vi "故障告警分析.vi"(8 "告警代码":u16, 9 "故障代码":u16, 10 "运行步序":u16, 11 "参数":string) -> (2 "报警内容":T1, 3 "简易报警状态":cluster{"故障状态":string, "报警状态":string})   [LabVIEW 2016, in "斯坦道氨氮.lvlib"]
panel:
  # "1、注射泵水样阀口堵塞；\n2、注射泵阀过载或丝杆无动作。"
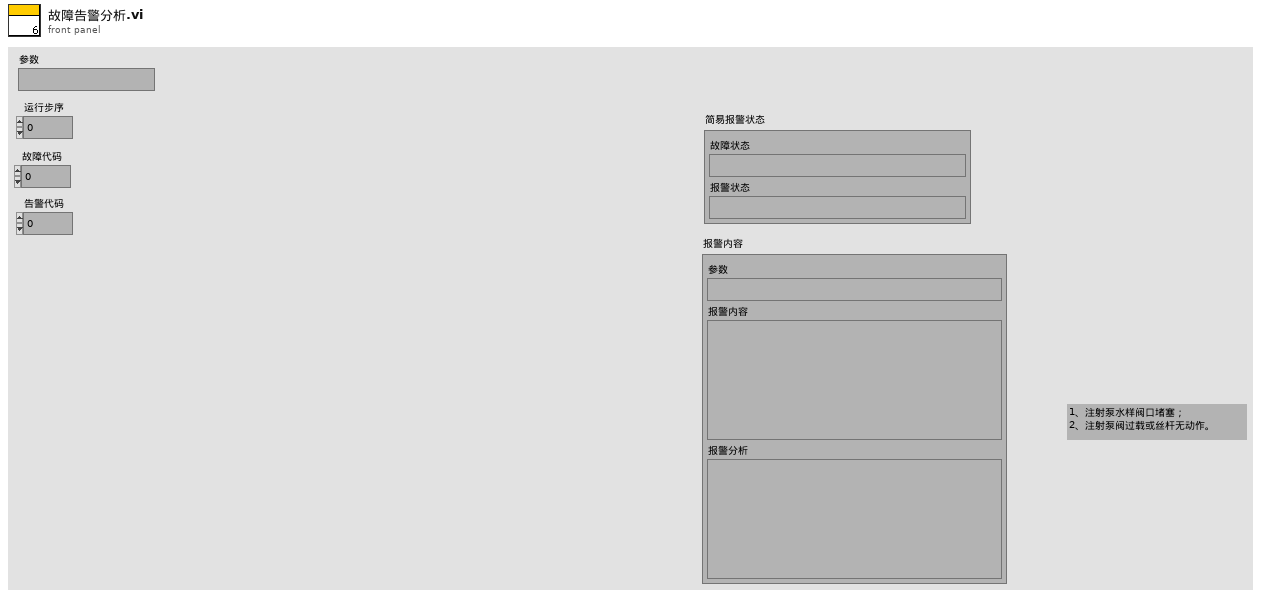
[diagram p1: front panel]
types:
  T1 = cluster{"参数":string, "报警内容":string, "报警分析":string}
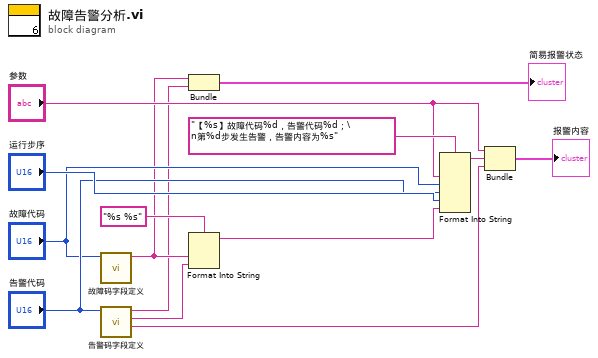
[diagram p0: block diagram]
diagram:
  n1 = call "故障码字段定义.vi"("故障代码"="故障代码") -> ("字符串"=w4:string)  [unwired: 10 in]
  n2 = call "告警码字段定义.vi"("告警代码"="告警代码") -> ("故障详情"=w1:string, "通用告警信息"=w2:string, "字符串"=w3:string)  [unwired: 8 in]
  n3 = Bundle("字符串"=w4, "字符串"=w3) -> (→"简易报警状态":cluster{"字符串":string, "字符串":string})  [unwired: 1 in]
  n4 = Format Into String(format string="%s %s" ("格式字符串"), w4, w2) -> (resulting string=w9:string)  [unwired: 2 in, 1 out]
  n5 = Format Into String(format string="【%s】故障代码%d，告警代码%d；\n第%d步发生告警，告警内容为%s" ("格式字符串"), "参数", "故障代码", "告警代码", "运行步序", w9) -> (resulting string=w7:string)  [unwired: 2 in, 1 out]
  n6 = Bundle("参数"="参数", w7, "故障详情"=w1) -> (→"报警内容":cluster{"参数":string, string, "故障详情":string})  [unwired: 1 in]
